vi "NorthWest Window Control.vi"() -> (0 "Error string":string)   [LabVIEW 2022 SP3]
uses:
  Anemometry/Anemometry Sub Vis/Globals/Dynamic_call_global.ph.vi
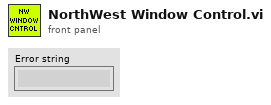
[diagram p1: front panel]
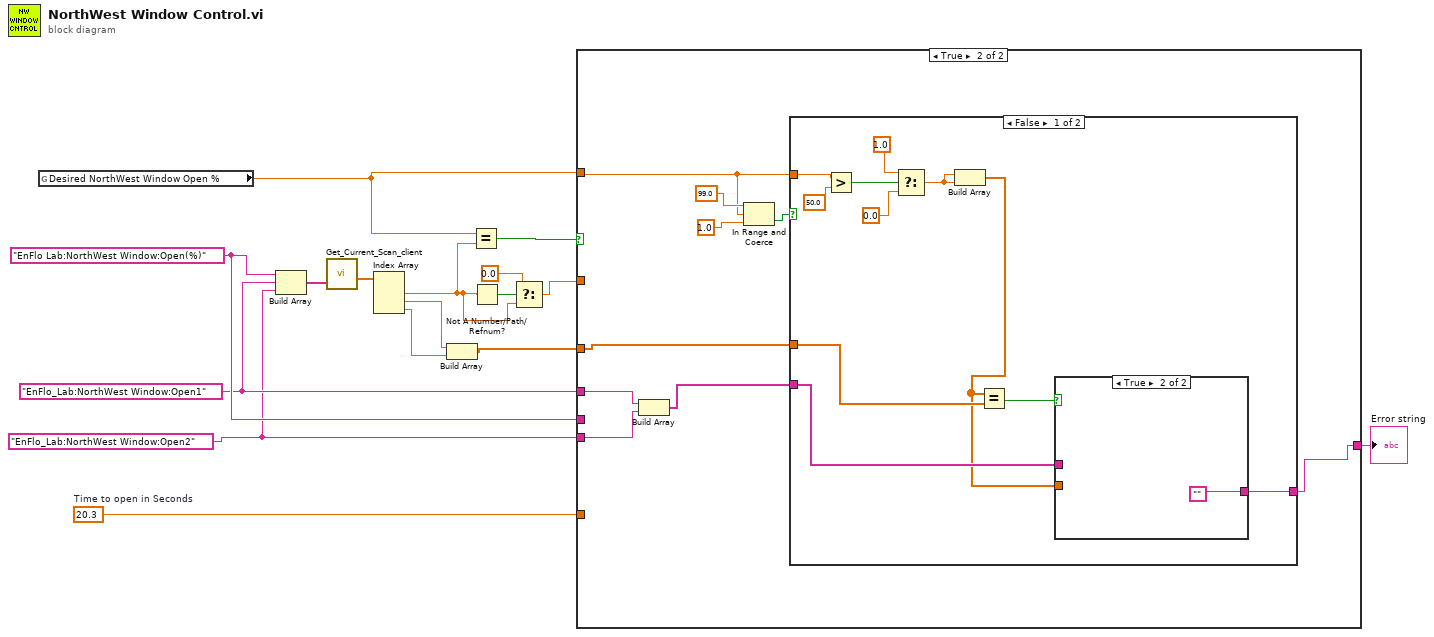
[diagram p0: block diagram]
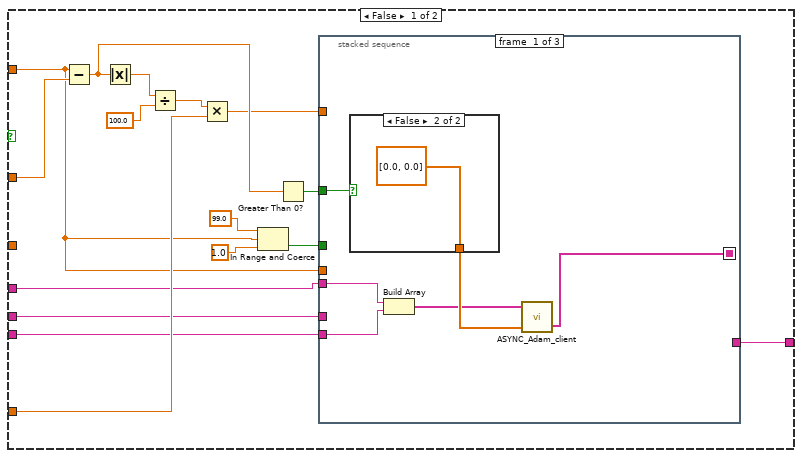
[diagram p2: hidden frame]
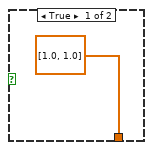
[diagram p3: hidden frame]
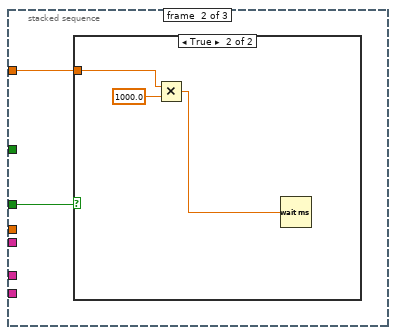
[diagram p4: hidden frame]
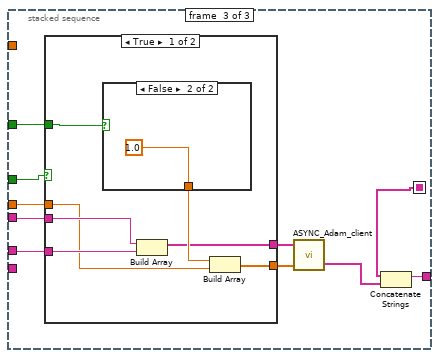
[diagram p6: hidden frame]
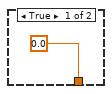
[diagram p7: hidden frame]
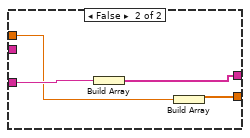
[diagram p8: hidden frame]
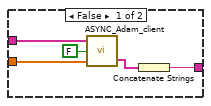
[diagram p9: hidden frame]
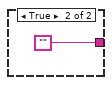
[diagram p10: hidden frame]
diagram:
  w4 = "EnFlo_Lab:NorthWest Window:Open2"
  w5 = "EnFlo_Lab:NorthWest Window:Open1"
  w13 = 20.3  # Time to open in Seconds
  w12 = "EnFlo Lab:NorthWest Window:Open(%)"
  n1 = global read "Dynamic_call_global.ph.vi" "Desired NorthWest Window Open %"() -> (w6:dbl)
  n2 = Build Array(w12, w5, w4) -> (w16:string[])
  n3 = call "Get_Current_Scan_client.vi"("multipleChannels"=w16) -> ("Numerical Values"=w15:dbl[])  [unwired: 1 in, 3 out]
  n4 = Index Array(array=w15) -> (element #1=w7:dbl, element #2=w3:dbl, element #3=w2:dbl)  [unwired: 3 in]
  n5 = Build Array(w3, w2) -> (w1:dbl[])
  n6 = Equal?(x=w6, y=w7) -> (x = y?=w14:bool)
  n7 = Not A Number/Path/Refnum?(number/path/refnum=w7) -> (NaN/Path/Refnum?=w10:bool)
  n8 = Select(t=0.0, s=w10, f=w7) -> (s? t:f=w9:dbl)
  n9 = case shown="True" w14 {
    tunnel: w6 -> [w23 w73]
    tunnel: w9 -> [w32 _]
    tunnel: w13 -> [w29 _]
    tunnel: w12 -> [w24 _]
    tunnel: [w22 w71] -> w11
    tunnel: w5 -> [w18 w69]
    tunnel: w4 -> [w17 w70]
    tunnel: w1 -> [_ w72]
    frame False {
      n10 = Subtract(x=w23, y=w32) -> (x-y=w27:dbl)
      n11 = Absolute Value(x=w27) -> (abs(x)=w28:dbl)
      n12 = Divide(x=w28, y=100.0) -> (x/y=w30:dbl)
      n13 = Multiply(x=w30, y=w29) -> (x*y=w25:dbl)
      n14 = In Range and Coerce(upper limit=99.0, x=w23, lower limit=1.0) -> (In Range?=w19:bool)  [unwired: 1 out]
      n15 = Greater Than 0?(x=w27) -> (x > 0?=w26:bool)
      n16 = stacked-sequence {
        seq-local: [w33 _ _] -> [_ _ w49]
        tunnel: w26 -> [w38 _ w55]
        tunnel: w25 -> [_ w42 _]
        tunnel: w18 -> [w36 _ w54]
        tunnel: w17 -> [w35 _ _]
        tunnel: w24 -> [_ _ w53]
        tunnel: w23 -> [_ _ w52]
        tunnel: [_ _ w46] -> w22
        tunnel: w19 -> [_ w41 w51]
        frame #0 {
          n17 = case shown="False" w38 {
            tunnel: [dbl[] [1.0, 1.0] ("Values") dbl[] [0.0, 0.0] ("Values")] -> w37
            frame True {
            }
            frame False {
            }
          }
          n18 = Build Array(w36, w35) -> (w34:string[])
          n19 = call "ASYNC_Adam_client.vi"("Values"=w37, "Channel Names"=w34) -> ("Scan Comments"=w33:string[])  [unwired: 1 in, 1 out]
        }
        frame #1 {
          n20 = case shown="True" w41 {
            tunnel: w42 -> [_ w45]
            frame False {
            }
            frame True {
              n21 = Multiply(x=w45, y=1000.0) -> (x*y=w43:dbl)
              n22 = Wait (ms)(milliseconds to wait=w43) -> ()  [unwired: 1 out]
            }
          }
        }
        frame #2 {
          n23 = case shown="True" w51 {
            tunnel: w55 -> [w62 _]
            tunnel: w54 -> [w61 _]
            tunnel: w53 -> [w59 w68]
            tunnel: w52 -> [w58 w67]
            tunnel: [w57 w66] -> w48
            tunnel: [w56 w65] -> w47
            frame True {
              n24 = case shown="False" w62 {
                tunnel: [0.0 1.0] -> w60
                frame True {
                }
                frame False {
                }
              }
              n25 = Build Array(w61, w59) -> (w57:string[])
              n26 = Build Array(w60, w58) -> (w56:dbl[])
            }
            frame False {
              n27 = Build Array(w68) -> (w66:string[])
              n28 = Build Array(w67) -> (w65:dbl[])
            }
          }
          n29 = call "ASYNC_Adam_client.vi"("Values"=w47, "Channel Names"=w48) -> ("Scan Comments"=w50:string[])  [unwired: 1 in, 1 out]
          n30 = Concatenate Strings(w49, w50) -> (w46:string)
        }
      }
    }
    frame True {
      n31 = Build Array(w69, w70) -> (w77:string[])
      n32 = In Range and Coerce(upper limit=99.0, x=w73, lower limit=1.0) -> (In Range?=w74:bool)  [unwired: 1 out]
      n33 = case shown="False" w74 {
        tunnel: w73 -> [w88 _]
        tunnel: w72 -> [w86 _]
        tunnel: w77 -> [w84 _]
        tunnel: [w79 ""] -> w71
        frame False {
          n34 = Greater?(x=w88, y=50.0) -> (0:w83:bool)
          n35 = Select(t=1.0, s=w83, f=0.0) -> (s? t:f=w78:dbl)
          n36 = Build Array(w78, w78) -> (w80:dbl[])
          n37 = Equal?(x=w80, y=w86) -> (x = y?=w85:bool)
          n38 = case shown="True" w85 {
            tunnel: w84 -> [w93 _]
            tunnel: w80 -> [w92 _]
            tunnel: [w89 ""] -> w79
            frame False {
              n39 = call "ASYNC_Adam_client.vi"("Values"=w92, "Check Value is in the scan table?"=FALSE, "Channel Names"=w93) -> ("Scan Comments"=w90:string[])  [unwired: 1 out]
              n40 = Concatenate Strings(w90) -> (w89:string)
            }
            frame True {
            }
          }
        }
        frame True {
        }
      }
    }
  }
  "Error string" <- w11
